vi "Medicao.View.vi"() -> ()   [LabVIEW 2019]
uses:
  Telas.ctl
  <vilib>/Utility/miscctls.llb/LVPositionTypeDef.ctl
  <vilib>/Utility/miscctls.llb/LVPointTypeDef.ctl
  TelaParametrosTeste/VariaveisParametros.vi
  Medicao/VariaveisMedicao.vi
  TelaConfig/Configuracao.Variaveis.vi
  Main/VariaveisTaskMedicao.vi
panel:
  in  "GraphCont":cluster{"X":dbl, "Y":dbl}[](graph)
  out "InfoContinuoRef":T1={"TempRampas"=0.0, "PicoMax"=0.0, "TextUnidMed"="segundos"}
  in  "GraphPontos":cluster{"X":dbl, "Y":dbl}[](array[cluster])
  in  "GraphSenoide":cluster{"X":dbl, "Y":dbl}[](array[cluster])
  out "TimeAquisicao":i32=1000
  out "TimeLastMed":u32
  out "TimeNowMed":u32
  out "Anemometro2":cluster{"X":dbl, "Y":dbl}[](graph)
  out "Anemometro1":cluster{"X":dbl, "Y":dbl}[](graph)
  out "CorrenteAero":cluster{"X":dbl, "Y":dbl}[](graph)
  out "ListaMedicoes":string[][](array[string])
  out "VelocidadeExaustor":cluster{"X":dbl, "Y":dbl}[](graph)
  out "TensaoAero":cluster{"X":dbl, "Y":dbl}[](graph)
  out "TimeInicio":u32
  out "TimeNow":u32
  out "TimeLast":u32
  out "ProximaTela":T2
  in  "Tab":enum32{"Page 1", "Page 2"}(tab)
  in  "QuantMonitora":T3(ring) caption="Tipos de Medição:"
  in  "TabTela":enum32{"Info", "Graph"}(tab)
  out "Text":string
  in  "TaxaTansmissãoDados":dbl caption="Taxa de transmissão de dados:"
  out "UnidadeTaxaTanmissãoDados":string
  out "GeracaoSelecionada":string
  in  "TabOndas":T4(tab)
  out "UnidadeRpm3":string
  in  "InfoContinuo":T1
  out "UnidadeSegundos2":string
  out "UnidadeRpm1":string
  out "UnidadeRpm2":string
  in  "InfoInSenoide":T5
  out "TaxaGeracao":dbl caption="Tempo entre pontos:"
  out "Pontos":dbl[](array[numeric]) caption="Pontos:"
  out "UnidadeSegundos1":string
  out "ListaMedicaoPorta":string[][](table)
  in  "TempoTeste":dbl caption="Tempo do teste:"
  out "UnidadeTempoTeste":string
  in  "MenosVeloz":bool
  in  "MaisVeloz":bool
  out "ValorGraph2":dbl format="%#_5g"
  out "ValorGraph":dbl format="%#_5g"
  out "Graph2":cluster{"X":dbl, "Y":dbl}[](graph)
  out "Graph":cluster{"X":dbl, "Y":dbl}[](graph)
  in  "TipoMedição":u16(ring) caption="Grafico de monitoramento" items=["Velocidade informada"=90, "Velocidade do motor"=91, "Anemômetro 1"=3, "Anemômetro 2"=4, "Corrente AeroGerador"=2, "Tensão AeroGerador"=1]
  in  "TipoMedição2":u16(ring) caption="Grafico de monitoramento" items=["Velocidade informada"=90, "Velocidade do motor"=91, "Anemômetro 1"=3, "Anemômetro 2"=4, "Corrente AeroGerador"=2, "Tensão AeroGerador"=1]
  in  "Play":bool
  in  "Stop":bool
  in  "Voltar":bool
  out "Info":string
  in  "BotaoProximaTela":bool
  in  "VoltarTela":bool
  in  "Salvar":bool
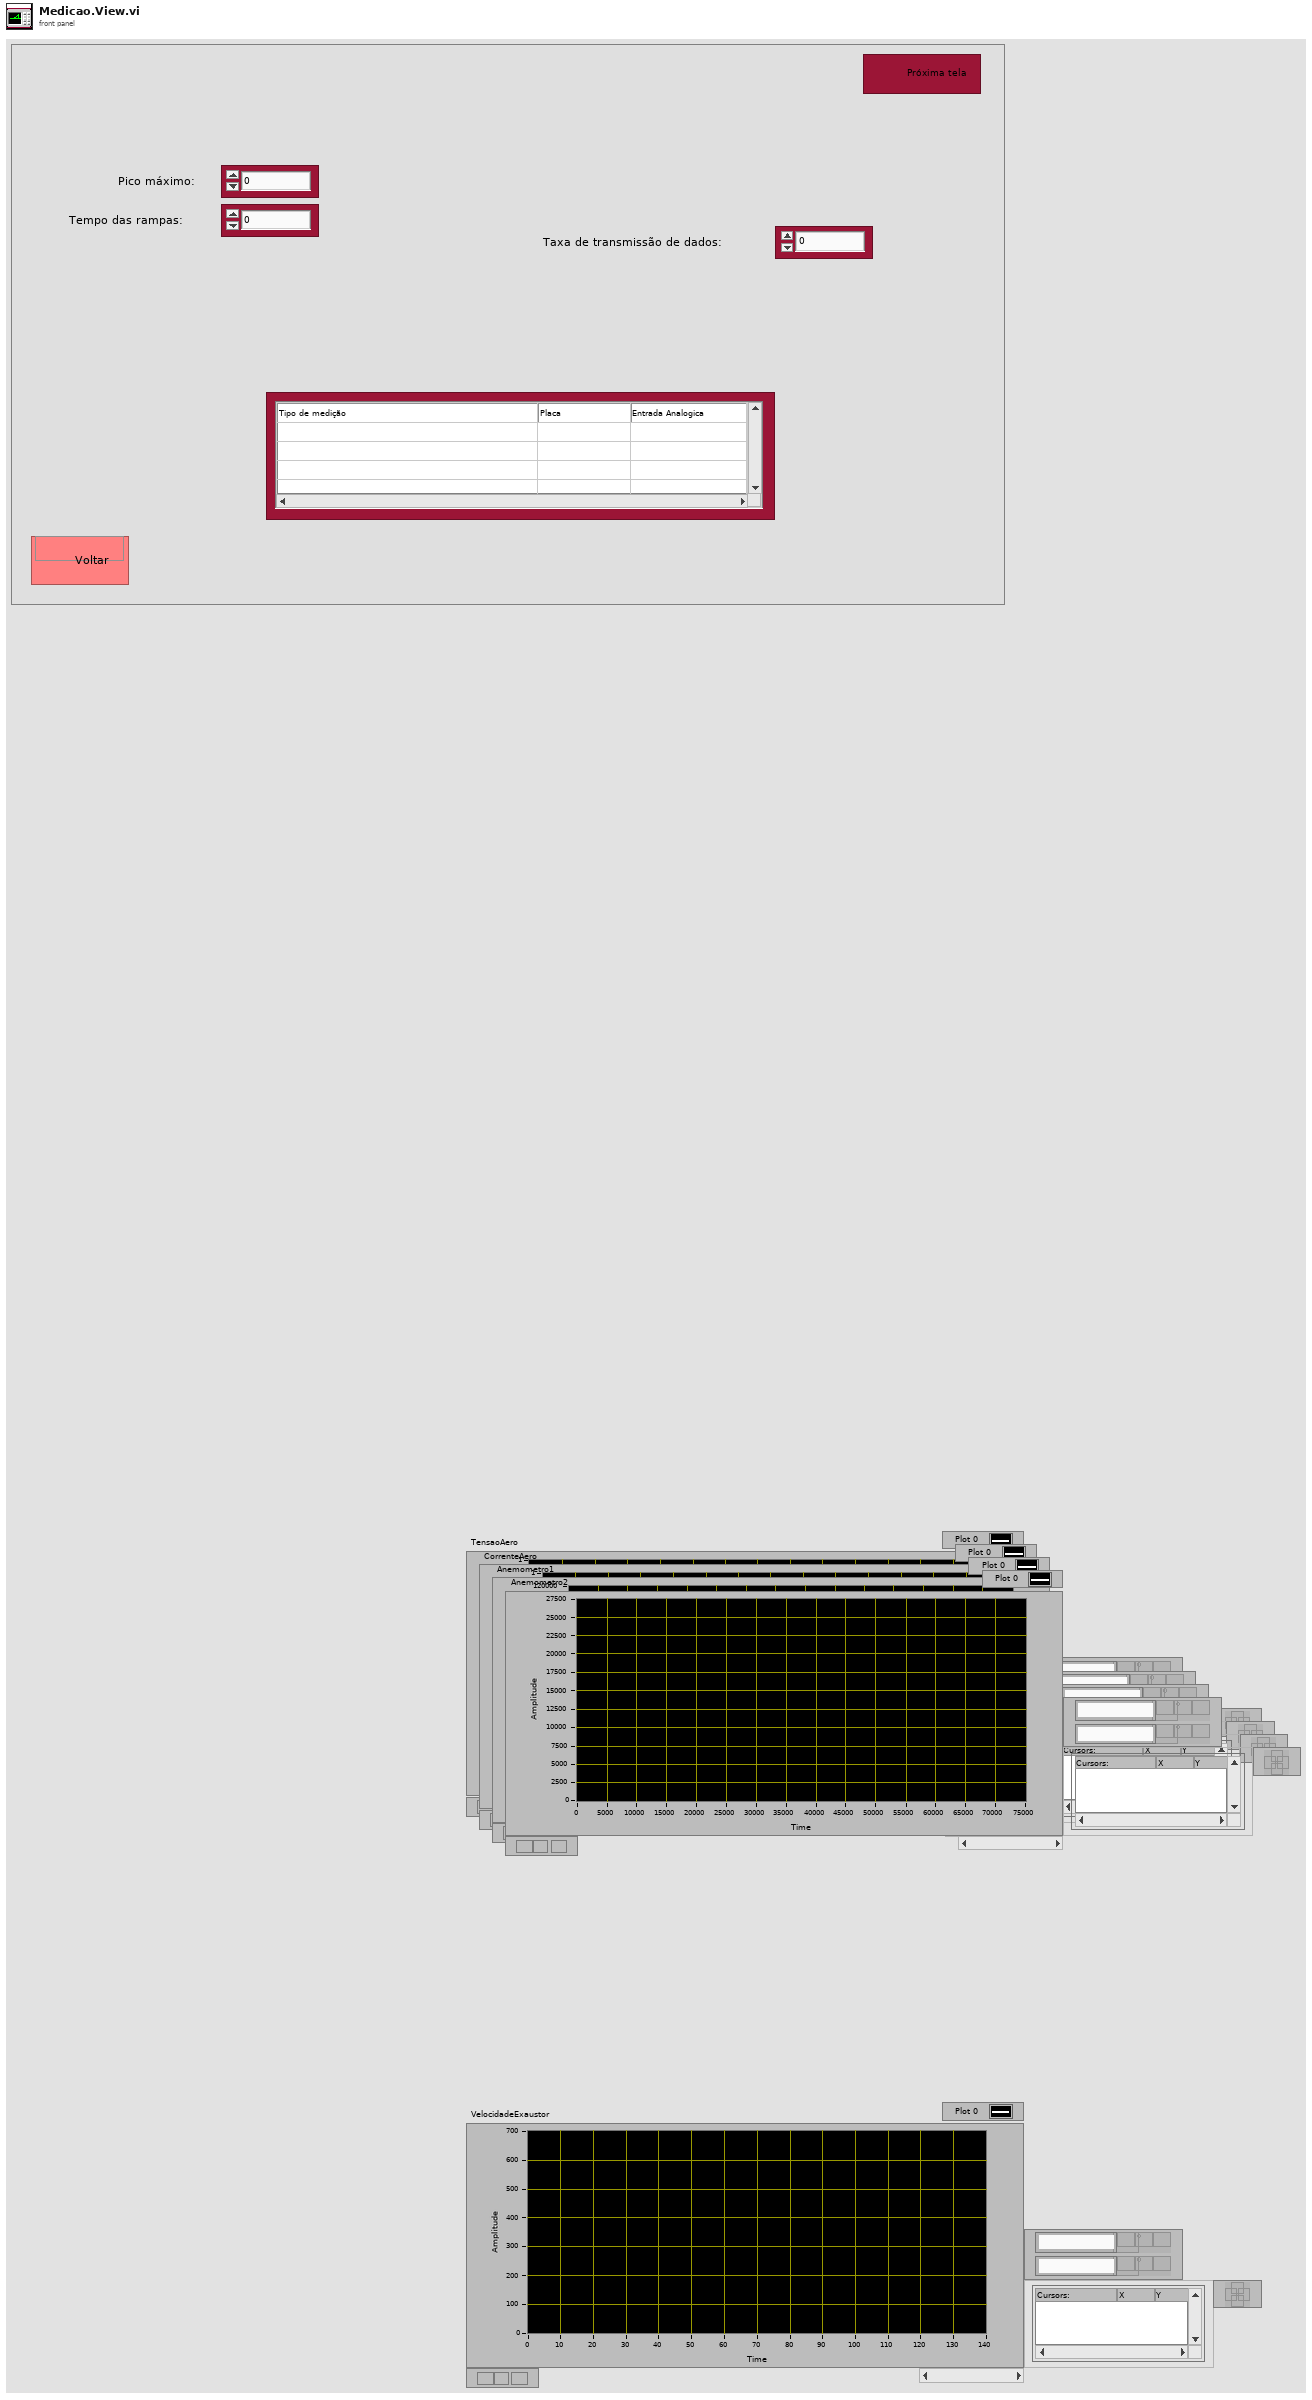
[diagram p1: front panel]
types:
  T1 = cluster{"TempRampas":dbl, "PicoMax":dbl, "TextUnidMed":string}
  T2 = typedef "Telas.ctl" = enum16{"Selecao", "Config", "Medicao", "ParametrosTeste"}
  T3 = enum16{"Monitorar um sinal", "Monitorar dois sinais"}
  T4 = enum32{"Contino", "Senoide", "Pontos", "Quadrada"}
  T5 = cluster{"PicoMax":dbl, "PicoMin":dbl, "RotacaoMinuto":dbl}
  T6 = typedef "LVPositionTypeDef.ctl" = cluster{"Left":i32, "Top":i32}
  T7 = typedef "LVPointTypeDef.ctl" = cluster{"Horizontal":i16, "Vertical":i16}
  T8 = enum16{"OndaContinua", "IniciarRotação", "StatusInversor", "FinalizarRotacao", "OndaSenoide", "OndaPontos", "VelocidadeExaustor"}
  T9 = enum16{"OndaContinua", "IniciarRotação", "StatusInversor", "FinalizarRotacao", "OndaSenoide", "OndaPontos"}
  T10 = enum16{"OndaContinua", "IniciarRotação", "StatusInversor", "FinalizarRotacao", "OndaSenoide", "OndaPontos", "VelocidadeExaustor", "SetInfInversor", "TempoAceleracao", "TempoDesaceleração"}
  T11 = cluster{"PicoRotacaoMax":dbl, "PicoRotacaoMin":dbl, "RotacoesMinuto":dbl}
  T12 = enum16{"None", "Continua", "Senoidal", "Quadrada"}
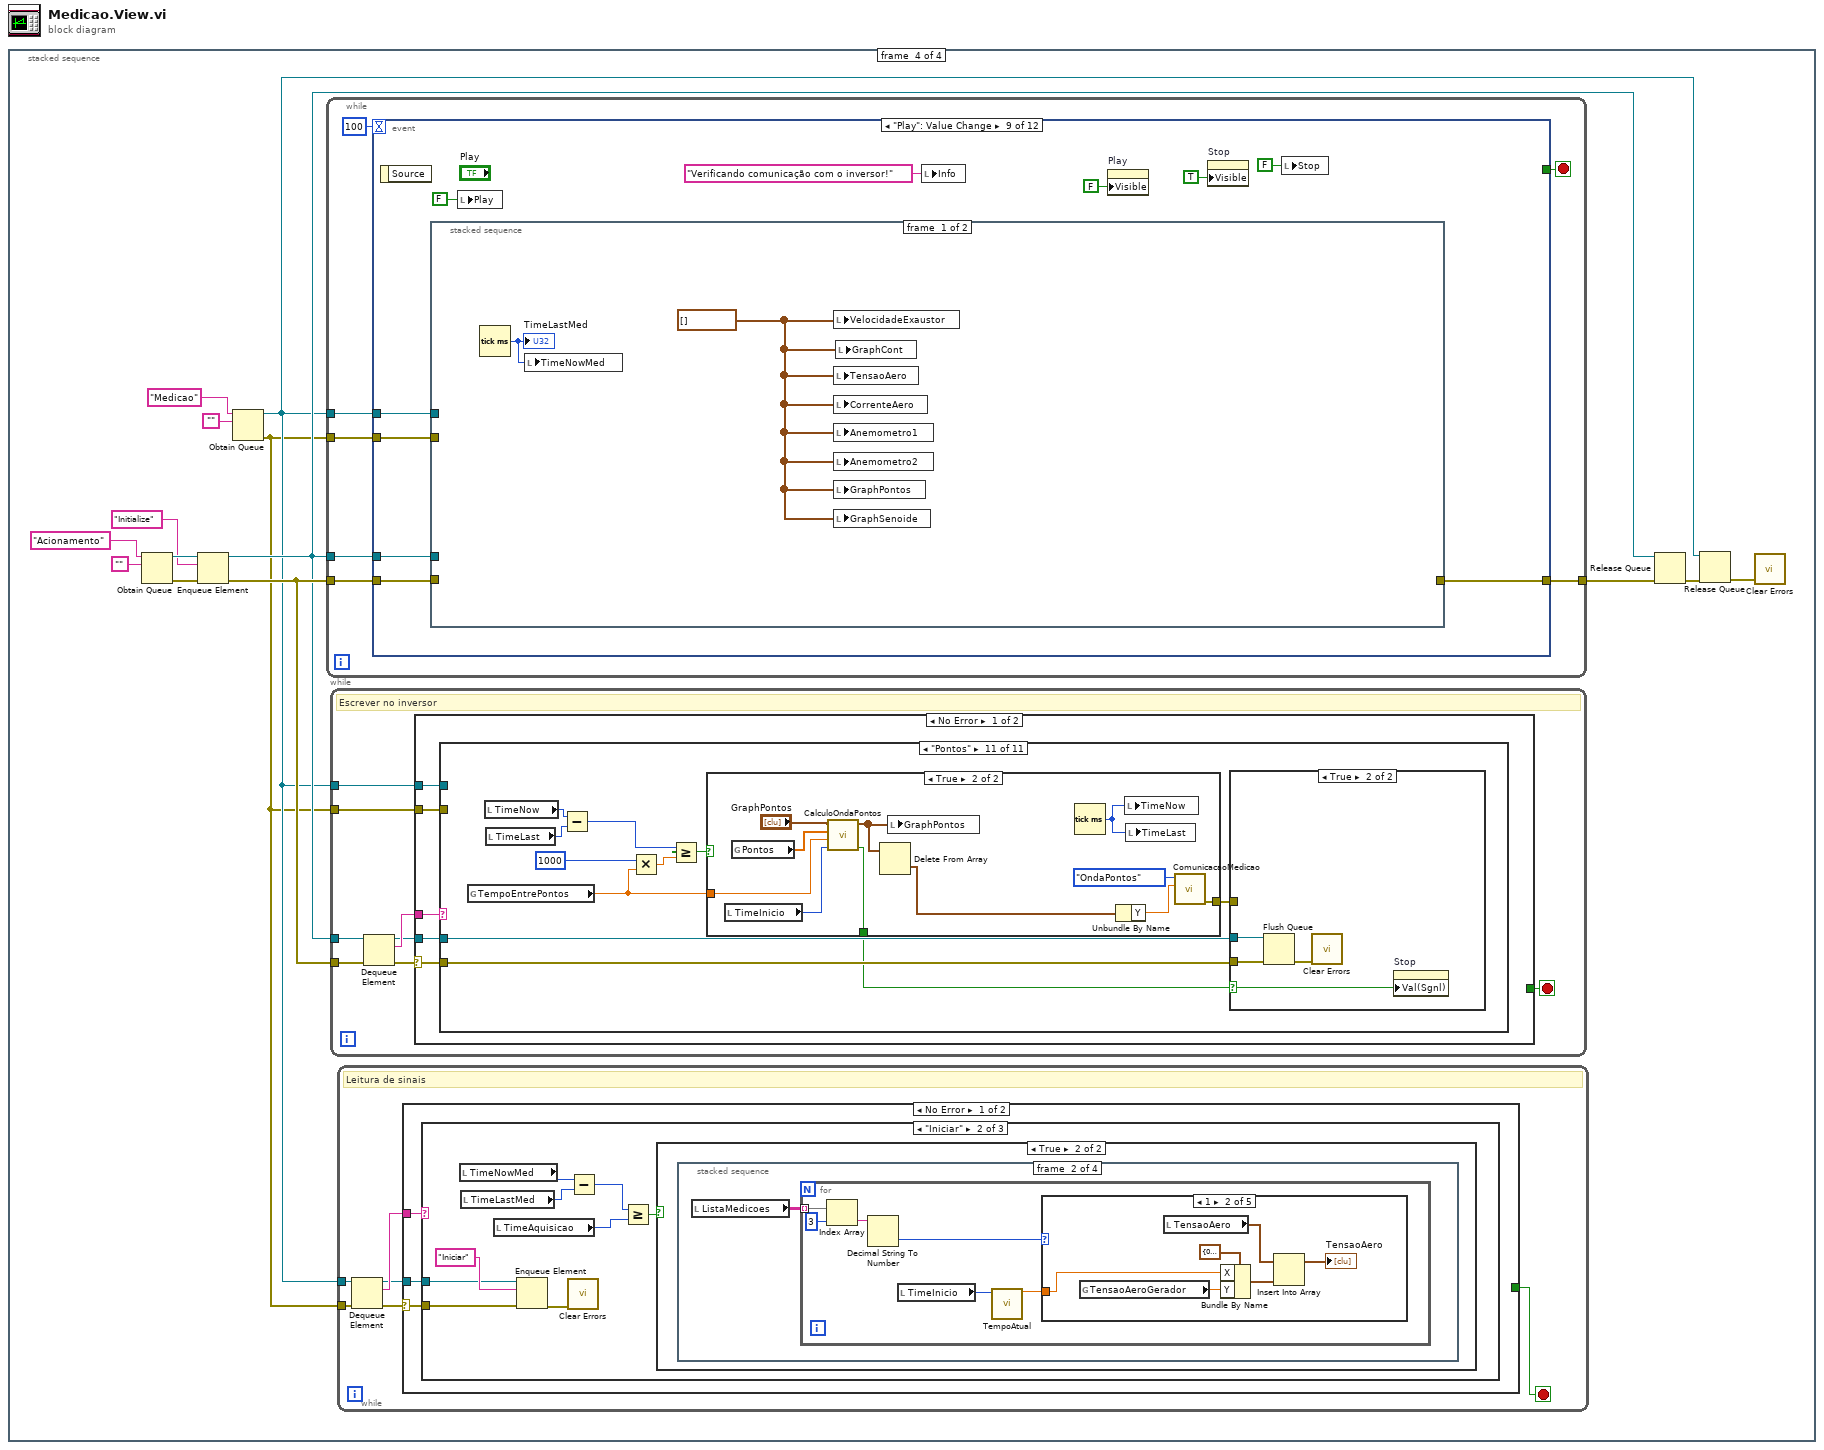
[diagram p0: block diagram]
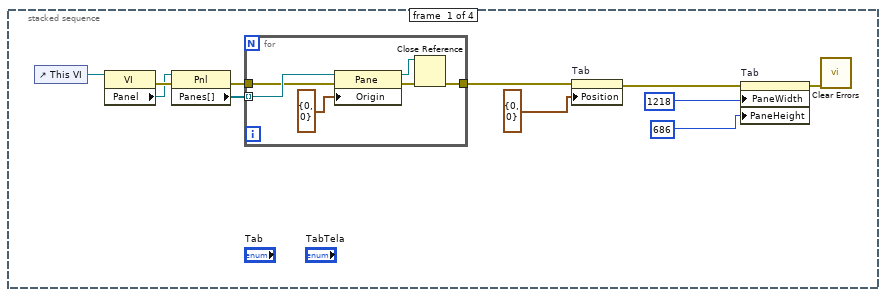
[diagram p2: hidden frame]
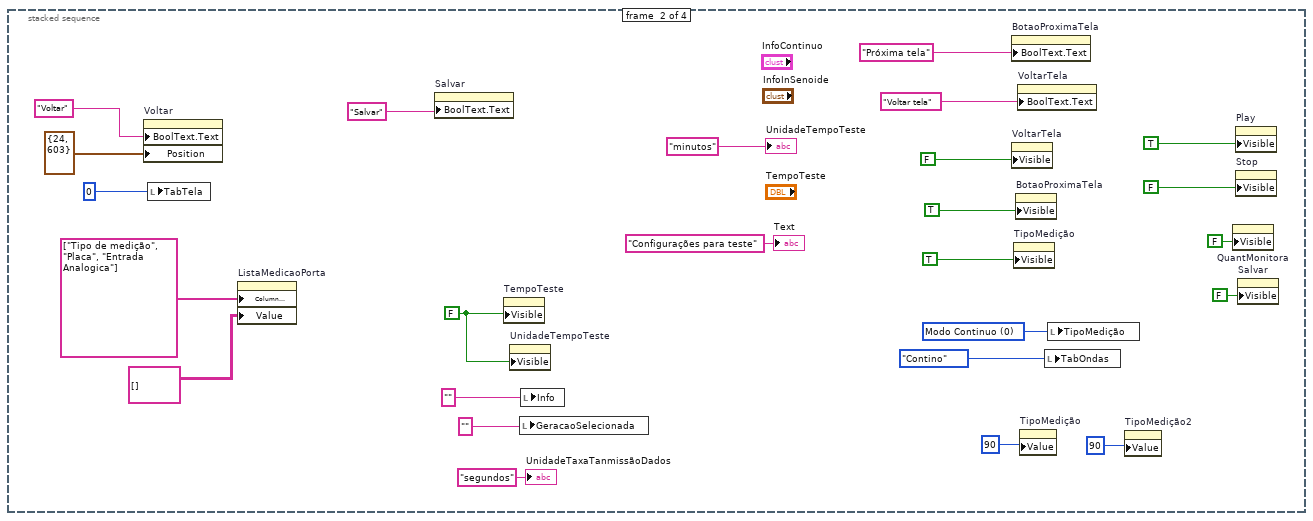
[diagram p3: hidden frame]
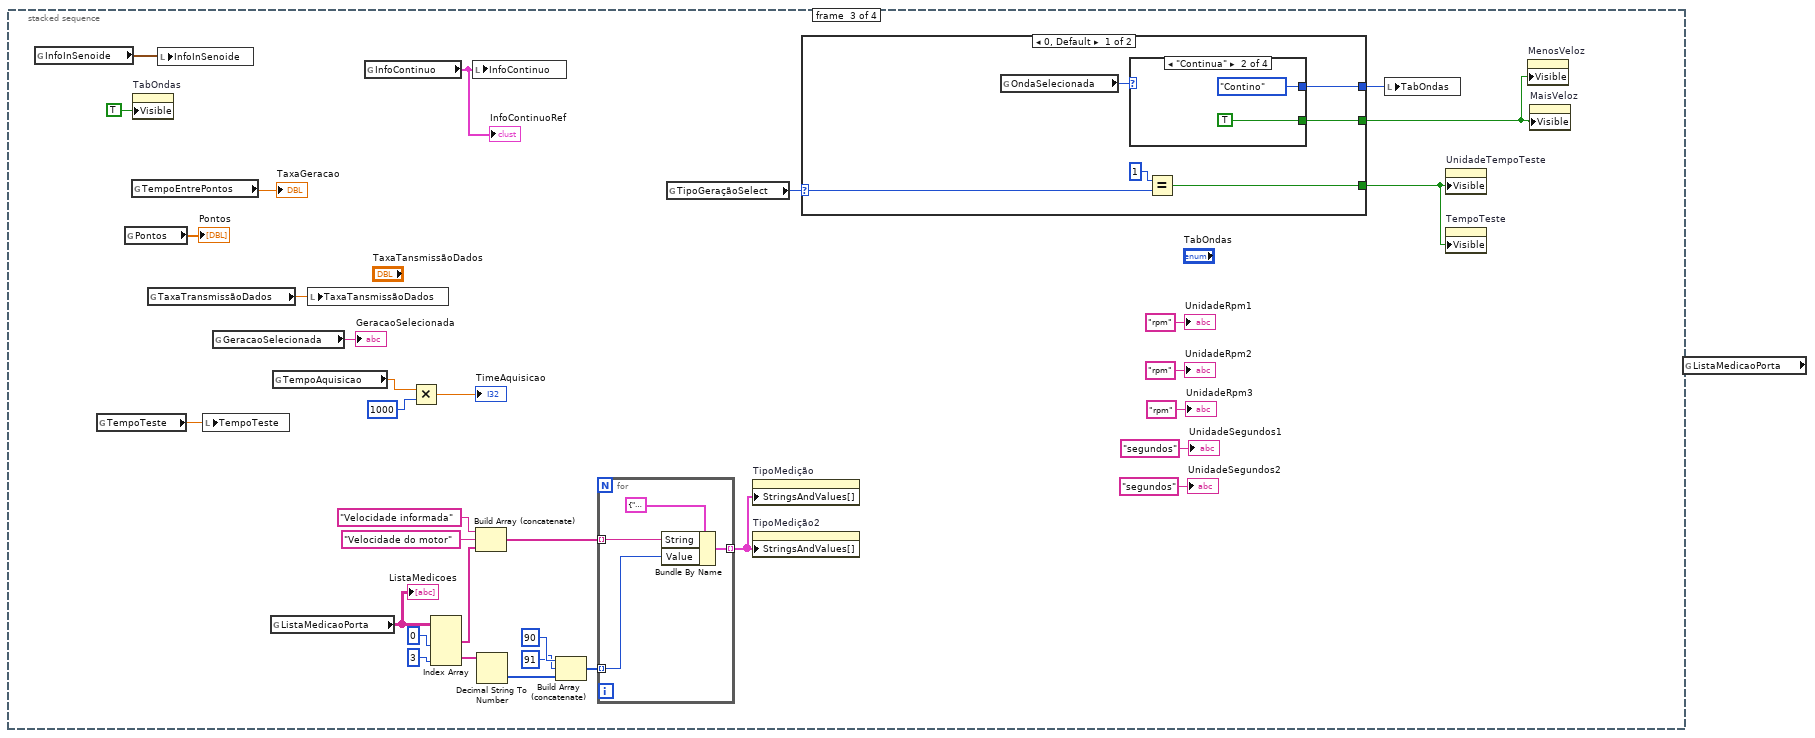
[diagram p4: hidden frame]
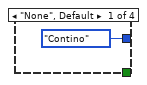
[diagram p5: hidden frame]
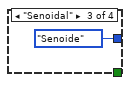
[diagram p6: hidden frame]
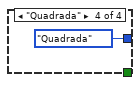
[diagram p7: hidden frame]
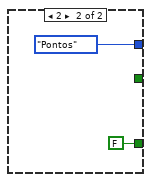
[diagram p8: hidden frame]
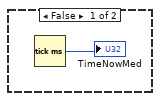
[diagram p10: hidden frame]
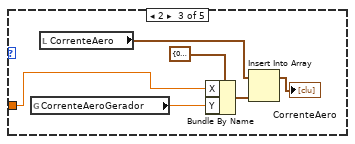
[diagram p13: hidden frame]
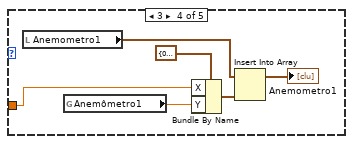
[diagram p14: hidden frame]
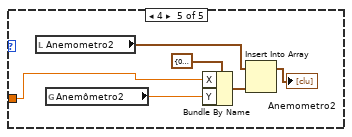
[diagram p15: hidden frame]
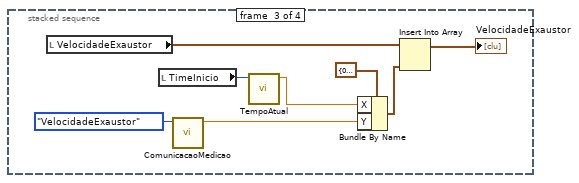
[diagram p16: hidden frame]
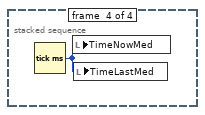
[diagram p17: hidden frame]
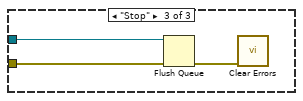
[diagram p18: hidden frame]
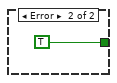
[diagram p19: hidden frame]
diagram:
  n1 = stacked-sequence {
    frame #0 {
      n2 = control-ref of="This VI"() -> (w8:refnum<vi>)
      n3 = property class="VI"(reference=w8) -> (error out=w11:errorcluster, "Panel"=w10:refnum<vi>)  [unwired: 1 in, 1 out]
      n4 = property class="Pnl"(reference=w10, error in=w11) -> (error out=w7:errorcluster, "Panes[]"=w9:refnum<vi>[])  [unwired: 1 out]
      n5 = for {
        tunnel: w9 -> [w17] mode=indexing
        tunnel: w7 -> [w13]
        tunnel: [w12] -> w6
        n6 = property class="Pane"(reference=w17, error in=w13, "Origin"=T7 {"Horizontal"=0, "Vertical"=0}) -> (reference out=w14:refnum<vi>, error out=w15:errorcluster)
        n7 = Close Reference(reference=w14, error in (no error)=w15) -> (error out=w12:errorcluster)
      }
      n8 = property on="Tab" class="TabCtl (strict)"(error in=w6, "Position"=T6 {"Left"=0, "Top"=0}) -> (error out=w5:errorcluster)  [unwired: 1 in, 1 out]
      n9 = property on="Tab" class="TabCtl (strict)"(error in=w5, "PaneWidth"=u32 1218 ("Tab Control Pane Dimension:Width"), "PaneHeight"=u32 686 ("Tab Control Pane Dimension:Height")) -> (error out=w4:errorcluster)  [unwired: 1 in, 1 out]
      n10 = call <vilib>:"Clear Errors.vi"("error in (no error)"=w4) -> ()  [unwired: 5 in, 2 out]
    }
    frame #1 {
      w26 = u16 0 items=["Modo Continuo", "Limitado por tempo", "Ponto por ponto"] ("SelecaoGeracao")
      w30 = FALSE
      n11 = property on="Voltar" class="Bool (strict)"("BoolText.Text"="Voltar" ("Boolean Text.Text"), "Position"=T6 {"Left"=24, "Top"=603}) -> ()  [unwired: 2 in, 2 out]
      n12 = local write "TabTela"(0) -> ()
      n13 = property on="ListaMedicaoPorta" class="Tbl (strict)"("Column Headers[]"=string[] ["Tipo de medição", "Placa", "Entrada Analogica"] ("Column Header Strings[]"), "Value"=string[][] [] ("Item Names")) -> ()  [unwired: 2 in, 2 out]
      n14 = property on="Salvar" class="Bool"("BoolText.Text"="Salvar" ("Boolean Text.Text")) -> ()  [unwired: 2 in, 2 out]
      n15 = property on="TempoTeste" class="DigNum (strict)"("Visible"=w30) -> ()  [unwired: 2 in, 2 out]
      n16 = property on="UnidadeTempoTeste" class="Str"("Visible"=w30) -> ()  [unwired: 2 in, 2 out]
      n17 = local write "GeracaoSelecionada"("" ("GeracaoSelecionada")) -> ()
      n18 = local write "Info"("" ("InfoConfig")) -> ()
      n19 = property on="BotaoProximaTela" class="Bool"("BoolText.Text"="Próxima tela" ("Boolean Text.Text")) -> ()  [unwired: 2 in, 2 out]
      n20 = property on="VoltarTela" class="Bool"("Visible"=FALSE) -> ()  [unwired: 2 in, 2 out]
      n21 = property on="TipoMedição" class="Ring (strict)"("Visible"=TRUE) -> ()  [unwired: 2 in, 2 out]
      n22 = property on="BotaoProximaTela" class="Bool"("Visible"=TRUE) -> ()  [unwired: 2 in, 2 out]
      n23 = property on="VoltarTela" class="Bool"("BoolText.Text"="Voltar tela" ("Boolean Text.Text")) -> ()  [unwired: 2 in, 2 out]
      n24 = property on="TipoMedição" class="Ring (strict)"("Value"=90) -> ()  [unwired: 2 in, 2 out]
      n25 = local write "TabOndas"(T4."Contino" ("TabOndas")) -> ()
      n26 = local write "TipoMedição"(w26) -> ()
      n27 = property on="TipoMedição2" class="Ring (strict)"("Value"=90) -> ()  [unwired: 2 in, 2 out]
      n28 = property on="QuantMonitora" class="Enum (strict)"("Visible"=FALSE) -> ()  [unwired: 2 in, 2 out]
      n29 = property on="Play" class="Bool (strict)"("Visible"=TRUE) -> ()  [unwired: 2 in, 2 out]
      n30 = property on="Stop" class="Bool (strict)"("Visible"=FALSE) -> ()  [unwired: 2 in, 2 out]
      n31 = property on="Salvar" class="Bool"("Visible"=FALSE) -> ()  [unwired: 2 in, 2 out]
      "UnidadeTempoTeste" <- "minutos" ("UnidadeTempoTeste")
      "UnidadeTaxaTanmissãoDados" <- "segundos" ("UnidadeTaxaTanmissãoDados")
      "Text" <- "Configurações para teste" ("String")
    }
    frame #2 {
      n32 = global read "VariaveisParametros.vi" "InfoInSenoide"() -> (w62:T11)
      n33 = global read "VariaveisParametros.vi" "TempoTeste"() -> (w72:dbl)
      n34 = global read "VariaveisParametros.vi" "Pontos"() -> (→"Pontos":dbl[])
      n35 = global read "VariaveisParametros.vi" "TempoEntrePontos"() -> (→"TaxaGeracao":dbl)
      n36 = property on="TabOndas" class="TabCtl (strict)"("Visible"=TRUE) -> ()  [unwired: 2 in, 2 out]
      n37 = global read "VariaveisParametros.vi" "TaxaTransmissãoDados"() -> (w64:dbl)
      n38 = local write "InfoInSenoide"(w62) -> ()
      n39 = local write "TempoTeste"(w72) -> ()
      n40 = global read "VariaveisParametros.vi" "GeracaoSelecionada"() -> (→"GeracaoSelecionada":string)
      n41 = global read "VariaveisParametros.vi" "ListaMedicaoPorta"() -> (w58:string[][])
      "ListaMedicoes" <- w58
      n42 = global read "VariaveisParametros.vi" "TempoAquisicao"() -> (w67:dbl)
      n43 = local write "TaxaTansmissãoDados"(w64) -> ()
      n44 = global read "VariaveisParametros.vi" "InfoContinuo"() -> (w73:T1)
      "InfoContinuoRef" <- w73
      n45 = Multiply(x=w67, y=1000) -> (x*y=→"TimeAquisicao":dbl)
      n46 = Index Array(array=w58, index (col) #1=0 ("disabled index (col)"), index (col) #2=3 ("index (col)")) -> (element #1=w59:string[], element #2=w57:string[])  [unwired: 2 in]
      n47 = local write "InfoContinuo"(w73) -> ()
      n48 = Build Array (concatenate)("Velocidade informada", "Velocidade do motor", w59) -> (w60:string[])
      n49 = Decimal String To Number(string=w57) -> (number=w56:i32[])  [unwired: 2 in, 1 out]
      n50 = Build Array (concatenate)(90, 91, w56) -> (w55:i32[])
      n51 = for {
        tunnel: w60 -> [w79] mode=indexing
        tunnel: [w78] -> w61 mode=indexing
        tunnel: w55 -> [w77] mode=indexing
        n52 = Bundle By Name(cluster=cluster{"String":string, "Value":u16} {"String"="Modo Continuo", "Value"=0}, "String"=w79, "Value"=w77) -> (w78:cluster{"String":string, "Value":u16})
      }
      n53 = global read "VariaveisParametros.vi" "TipoGeraçãoSelect"() -> (w76:u16)
      n54 = property on="TipoMedição" class="Ring (strict)"("StringsAndValues[]"=w61) -> ()  [unwired: 2 in, 2 out]
      n55 = property on="TipoMedição2" class="Ring (strict)"("StringsAndValues[]"=w61) -> ()  [unwired: 2 in, 2 out]
      n56 = case shown="0, Default" w76 {
        selector: w76 -> [w84 _]
        tunnel: [w85 T4."Pontos" ("TabOndas")] -> w75
        tunnel: [w82 FALSE] -> w63
        tunnel: [w81 _] -> w48
        frame 0, Default {
          n57 = global read "VariaveisParametros.vi" "OndaSelecionada"() -> (w86:T12)
          n58 = case shown="\"Continua\"" w86 {
            tunnel: [T4."Contino" ("TabOndas") T4."Contino" ("TabOndas") T4."Senoide" ("TabOndas") T4."Quadrada" ("TabOndas")] -> w85
            tunnel: [_ TRUE _ _] -> w81
            frame "None", Default {
            }
            frame "Continua" {
            }
            frame "Senoidal" {
            }
            frame "Quadrada" {
            }
          }
          n59 = Equal?(x=u16 1, y=w84) -> (x = y?=w82:bool)
        }
        frame 2 {
        }
      }
      n60 = local write "TabOndas"(w75) -> ()
      n61 = property on="UnidadeTempoTeste" class="Str"("Visible"=w63) -> ()  [unwired: 2 in, 2 out]
      n62 = property on="TempoTeste" class="DigNum (strict)"("Visible"=w63) -> ()  [unwired: 2 in, 2 out]
      n63 = property on="MenosVeloz" class="Bool (strict)"("Visible"=w48) -> ()  [unwired: 2 in, 2 out]
      n64 = property on="MaisVeloz" class="Bool (strict)"("Visible"=w48) -> ()  [unwired: 2 in, 2 out]
      n65 = global read "VariaveisParametros.vi" "ListaMedicaoPorta"() -> (→"ListaMedicaoPorta":string[][])
      "UnidadeRpm3" <- "rpm" ("UnidadeTaxaTanmissãoDados 3")
      "UnidadeRpm2" <- "rpm" ("UnidadeTaxaTanmissãoDados 4")
      "UnidadeRpm1" <- "rpm" ("UnidadeTaxaTanmissãoDados 5")
      "UnidadeSegundos1" <- "segundos" ("UnidadeTaxaTanmissãoDados 6")
      "UnidadeSegundos2" <- "segundos" ("UnidadeTaxaTanmissãoDados 2")
    }
    frame #3 {
      n66 = Obtain Queue(name (unnamed)="Acionamento", element data type="") -> (queue out=w105:refnum<queue>, error out=w106:errorcluster)  [unwired: 3 in, 1 out]
      n67 = Enqueue Element(queue=w105, element="Initialize", error in (no error)=w106) -> (queue out=w100:refnum<queue>, error out=w101:errorcluster)  [unwired: 1 in, 1 out]
      n68 = Obtain Queue(name (unnamed)="Medicao", element data type="") -> (queue out=w95:refnum<queue>, error out=w94:errorcluster)  [unwired: 3 in, 1 out]
      n69 = while {
        tunnel: w100 -> [w401]
        tunnel: [w400] -> w102
        tunnel: w101 -> [w399]
        tunnel: w95 -> [w398]
        tunnel: w94 -> [w397]
        stop <- w402 stop-if-true
        n70 = event shown="[8] \"Play\": Value Change" {
          selector: _ -> [_ _ _ _ _ _ _ _ _ _ _ _]
          dyn-events: _ -> [_ _ _ _ _ _ _ _ _ _ _ _]
          timeout: 100 -> [_ _ _ _ _ _ _ _ _ _ _ _]
          tunnel: [FALSE TRUE _ _ _ _ _ _ _ _ _ _] -> w402
          tunnel: w401 -> [_ _ _ _ _ _ _ _ w532 w581 w599 w619]
          tunnel: [w404 _ _ _ _ _ _ _ w534 _ w598 w618] -> w400
          tunnel: w399 -> [w404 _ _ _ _ _ _ _ w533 w580 w600 w620]
          tunnel: w398 -> [_ _ _ _ _ _ _ _ w529 _ _ _]
          tunnel: w397 -> [_ _ _ _ _ _ _ _ w530 _ _ _]
          event Timeout {
            n71 = event-data() -> ()  [unwired: 1 in, 3 out]
            n72 = local read "TabTela"() -> (w405:enum32{"Info", "Graph"})
            n73 = case shown="\"Graph\"" w405 {
              frame Default {
              }
              frame "Graph" {
                n74 = property on="TipoMedição" class="Ring (strict)"() -> ("Value"=w439:u16)  [unwired: 2 in, 2 out]
                n75 = case shown="3" w439 {
                  tunnel: [cluster{"X":dbl, "Y":dbl}[] [] ("OndaCont") w444 w454 w456 w458 w460 w462] -> w437
                  tunnel: ["" w442 "RPM" "Volts" "Ampere" "Velocidade (m/s)" "Velocidade (m/s)"] -> w438
                  frame Default {
                  }
                  frame 90 {
                    n76 = local read "TabOndas"() -> (w443:T4)
                    n77 = case shown="\"Senoide\"" w443 {
                      tunnel: [cluster{"X":dbl, "Y":dbl}[] [] ("OndaCont") w447 w450 w452] -> w444
                      tunnel: ["" "RPM" "RPM" "RPM"] -> w442
                      frame Default {
                      }
                      frame "Contino" {
                        n78 = local read "VelocidadeExaustor"() -> (w447:cluster{"X":dbl, "Y":dbl}[])
                      }
                      frame "Senoide" {
                        n79 = local read "GraphSenoide"() -> (w450:cluster{"X":dbl, "Y":dbl}[])
                      }
                      frame "Pontos" {
                        n80 = local read "GraphPontos"() -> (w452:cluster{"X":dbl, "Y":dbl}[])
                      }
                    }
                  }
                  frame 91 {
                    n81 = local read "VelocidadeExaustor"() -> (w454:cluster{"X":dbl, "Y":dbl}[])
                  }
                  frame 1 {
                    n82 = local read "TensaoAero"() -> (w456:cluster{"X":dbl, "Y":dbl}[])
                  }
                  frame 2 {
                    n83 = local read "CorrenteAero"() -> (w458:cluster{"X":dbl, "Y":dbl}[])
                  }
                  frame 3 {
                    n84 = local read "Anemometro1"() -> (w460:cluster{"X":dbl, "Y":dbl}[])
                  }
                  frame 4 {
                    n85 = local read "Anemometro2"() -> (w462:cluster{"X":dbl, "Y":dbl}[])
                  }
                }
                "Graph" <- w437
                n86 = property on="Graph" class="XYGraph (strict)"("YScale.NameLbl.Text"=w438) -> ()  [unwired: 2 in, 2 out]
                n87 = Delete From Array(array=w437) -> (deleted portion=w436:cluster{"X":dbl, "Y":dbl})  [unwired: 2 in, 1 out]
                n88 = Unbundle By Name(w436) -> ("Y"=→"ValorGraph":dbl)
              }
            }
            n89 = case shown="\"Graph\"" w405 {
              frame Default {
              }
              frame "Graph" {
                n90 = property on="TipoMedição2" class="Ring (strict)"() -> ("Value"=w410:u16)  [unwired: 2 in, 2 out]
                n91 = case shown="4" w410 {
                  tunnel: [cluster{"X":dbl, "Y":dbl}[] [] ("OndaCont") w416 w426 w428 w430 w432 w434] -> w409
                  tunnel: ["" w414 "RPM" "Volts" "Ampere" "Velocidade (m/s)" "Velocidade (m/s)"] -> w408
                  frame Default {
                  }
                  frame 90 {
                    n92 = local read "TabOndas"() -> (w415:T4)
                    n93 = case shown="\"Senoide\"" w415 {
                      tunnel: [cluster{"X":dbl, "Y":dbl}[] [] ("OndaCont") w419 w422 w424] -> w416
                      tunnel: ["" "RPM" "RPM" "RPM"] -> w414
                      frame Default {
                      }
                      frame "Contino" {
                        n94 = local read "VelocidadeExaustor"() -> (w419:cluster{"X":dbl, "Y":dbl}[])
                      }
                      frame "Senoide" {
                        n95 = local read "GraphSenoide"() -> (w422:cluster{"X":dbl, "Y":dbl}[])
                      }
                      frame "Pontos" {
                        n96 = local read "GraphPontos"() -> (w424:cluster{"X":dbl, "Y":dbl}[])
                      }
                    }
                  }
                  frame 91 {
                    n97 = local read "VelocidadeExaustor"() -> (w426:cluster{"X":dbl, "Y":dbl}[])
                  }
                  frame 1 {
                    n98 = local read "TensaoAero"() -> (w428:cluster{"X":dbl, "Y":dbl}[])
                  }
                  frame 2 {
                    n99 = local read "CorrenteAero"() -> (w430:cluster{"X":dbl, "Y":dbl}[])
                  }
                  frame 3 {
                    n100 = local read "Anemometro1"() -> (w432:cluster{"X":dbl, "Y":dbl}[])
                  }
                  frame 4 {
                    n101 = local read "Anemometro2"() -> (w434:cluster{"X":dbl, "Y":dbl}[])
                  }
                }
                "Graph2" <- w409
                n102 = Delete From Array(array=w409) -> (deleted portion=w411:cluster{"X":dbl, "Y":dbl})  [unwired: 2 in, 1 out]
                n103 = property on="Graph2" class="XYGraph (strict)"("YScale.NameLbl.Text"=w408) -> ()  [unwired: 2 in, 2 out]
                n104 = Unbundle By Name(w411) -> ("Y"=→"ValorGraph2":dbl)
              }
            }
          }
          event "Voltar": Value Change {
            n105 = event-data() -> ()  [unwired: 1 in, 6 out]
            n106 = local write "Voltar"(FALSE ("VoltarButton")) -> ()
            n107 = local write "TabTela"(enum32{"Info", "Graph"}."Info" ("TabTela")) -> ()
            "ProximaTela" <- Telas."Selecao" ("NextScreen")
          }
          event "Salvar": Value Change {
            n108 = event-data() -> ()  [unwired: 1 in, 1 out]
            n109 = stacked-sequence {
              seq-local: [w469 _] -> [_ w482]
              frame #0 {
                # "Verifica se o campo esta preenchido corretamente"
                n110 = for {
                  N: 20 -> [_]
                  tunnel: [w470] -> w468 mode=indexing
                  i -> [w471]
                  n111 = case shown="1" w471 {
                    tunnel: [TRUE TRUE] -> w470
                    frame 0, Default {
                    }
                    frame 1 {
                      n112 = local read "VelocidadeExaustor"() -> (w474:cluster{"X":dbl, "Y":dbl}[])
                      n113 = local read "GraphPontos"() -> (w480:cluster{"X":dbl, "Y":dbl}[])
                      n114 = local read "GraphSenoide"() -> (w479:cluster{"X":dbl, "Y":dbl}[])
                      n115 = global write "VariaveisMedicao.vi" "VelocidadeExaustor"(w474) -> ()
                      n116 = global write "VariaveisMedicao.vi" "GraphSenoide"(w479) -> ()
                      n117 = global write "VariaveisMedicao.vi" "GraphPontos"(w480) -> ()
                      n118 = global write "VariaveisMedicao.vi" "OndaCont"("GraphCont") -> ()
                      n119 = local read "TensaoAero"() -> (w478:cluster{"X":dbl, "Y":dbl}[])
                      n120 = local read "CorrenteAero"() -> (w477:cluster{"X":dbl, "Y":dbl}[])
                      n121 = local read "Anemometro1"() -> (w476:cluster{"X":dbl, "Y":dbl}[])
                      n122 = local read "Anemometro2"() -> (w475:cluster{"X":dbl, "Y":dbl}[])
                      n123 = global write "VariaveisMedicao.vi" "Anemometro1"(w476) -> ()
                      n124 = global write "VariaveisMedicao.vi" "Anemometro1"(w475) -> ()
                      n125 = global write "VariaveisMedicao.vi" "CorrenteAero"(w477) -> ()
                      n126 = global write "VariaveisMedicao.vi" "TensaoAero"(w478) -> ()
                    }
                  }
                }
                n127 = And Array Elements(Boolean array=w468) -> (logical AND=w469:bool)
              }
              frame #1 {
                n128 = case shown="True" w482 {
                  frame False {
                    # "Algo não esta preenchido corretamente"
                    "Info" <- "" ("InfoConfig")
                  }
                  frame True {
                    # "Preenchimento correto dos campos"
                    n129 = call "SalvarInformacoesRelatorio.vi"() -> ("error out"=w485:errorcluster, "NomeDocumento"=w484:string)  [unwired: 10 in]
                    n130 = case shown="No Error" w485 {
                      selector: w485 -> [w489 _]
                      tunnel: [w490 "Erro ao salvar as variavies" ("InfoConfig")] -> w486
                      tunnel: w484 -> [w488 _]
                      frame No Error {
                        n131 = call "Geracao_Excel.vi"("error in (no error)"=w489, "FileName"=w488) -> ("error out"=w487:errorcluster)  [unwired: 9 in]
                        n132 = case shown="Error .." w487 {
                          tunnel: ["Informações salvas e gerado relatório" ("InfoConfig") "Informações salvas e erro ao gerar o relatório" ("InfoConfig")] -> w490
                          frame No Error {
                          }
                          frame Error {
                          }
                        }
                      }
                      frame Error {
                      }
                    }
                    n133 = local write "Info"(w486) -> ()
                  }
                }
              }
            }
          }
          event "BotaoProximaTela": Value Change {
            n134 = event-data() -> ()  [unwired: 1 in, 1 out]
            n135 = local read "TabTela"() -> (w499:enum32{"Info", "Graph"})
            n136 = Increment(x=w499) -> (x+1=w495:enum32{"Info", "Graph"})
            n137 = case shown="\"Info\"" w495 {
              tunnel: [TRUE FALSE TRUE] -> w498
              tunnel: [TRUE TRUE FALSE] -> w497
              tunnel: [TRUE FALSE TRUE] -> w496
              frame Default {
              }
              frame "Info" {
                w503 = u16 0 ("Value (Signaling)")
                n138 = property on="TipoMedição" class="Ring (strict)"("Val(Sgnl)"=w503) -> ()  [unwired: 2 in, 2 out]
                n139 = property on="TipoMedição2" class="Ring (strict)"("Value"=w503) -> ()  [unwired: 2 in, 2 out]
              }
              frame "Graph" {
              }
            }
            n140 = local write "TabTela"(w495) -> ()
            n141 = property on="Salvar" class="Bool"("Visible"=TRUE) -> ()  [unwired: 2 in, 2 out]
            n142 = property on="VoltarTela" class="Bool"("Visible"=w498) -> ()  [unwired: 2 in, 2 out]
            n143 = property on="ProximaTela" class="Bool"("Visible"=w497) -> ()  [unwired: 2 in, 2 out]
            n144 = property on="TipoMedição" class="Ring (strict)"("Visible"=w496) -> ()  [unwired: 2 in, 2 out]
          }
          event "VoltarTela": Value Change {
            n145 = event-data() -> ()  [unwired: 1 in, 6 out]
            n146 = local read "TabTela"() -> (w515:enum32{"Info", "Graph"})
            n147 = property on="Salvar" class="Bool"("Visible"=FALSE) -> ()  [unwired: 2 in, 2 out]
            n148 = Decrement(x=w515) -> (x-1=w511:enum32{"Info", "Graph"})
            n149 = local write "TabTela"(w511) -> ()
            n150 = case shown="Default" w511 {
              tunnel: [TRUE FALSE TRUE] -> w514
              tunnel: [TRUE TRUE FALSE] -> w513
              tunnel: [TRUE FALSE TRUE] -> w512
              frame Default {
              }
              frame "Info" {
              }
              frame "Graph" {
              }
            }
            n151 = property on="VoltarTela" class="Bool"("Visible"=w514) -> ()  [unwired: 2 in, 2 out]
            n152 = property on="ProximaTela" class="Bool"("Visible"=w513) -> ()  [unwired: 2 in, 2 out]
            n153 = property on="TipoMedição" class="Ring (strict)"("Visible"=w512) -> ()  [unwired: 2 in, 2 out]
          }
          event "TipoMedição": Value Change {
            n154 = event-data() -> ()  [unwired: 1 in, 1 out]
          }
          event "TipoMedição2": Value Change {
            n155 = event-data() -> ()  [unwired: 1 in, 1 out]
          }
          event "QuantMonitora": Value Change {
            n156 = event-data() -> ()  [unwired: 1 in, 6 out]
            n157 = case shown="\"Monitorar dois sinais\"" "QuantMonitora" {
              tunnel: [FALSE TRUE] -> w525
              frame "Monitorar um sinal", Default {
              }
              frame "Monitorar dois sinais" {
              }
            }
            n158 = property on="TipoMedição2" class="Ring (strict)"("Visible"=w525) -> ()  [unwired: 2 in, 2 out]
          }
          event "Play": Value Change {
            n159 = event-data() -> ()  [unwired: 1 in, 1 out]
            n160 = stacked-sequence {
              tunnel: [_ w555] -> w534
              tunnel: w533 -> [_ w554]
              tunnel: w532 -> [_ w553]
              tunnel: w530 -> [_ w551]
              tunnel: w529 -> [_ w550]
              frame #0 {
                w539 = cluster{"X":dbl, "Y":dbl}[] [] ("OndaCont")
                n161 = Tick Count (ms)() -> (millisecond timer value=w540:u32)
                "TimeLastMed" <- w540
                n162 = local write "TimeNowMed"(w540) -> ()
                n163 = local write "VelocidadeExaustor"(w539) -> ()
                n164 = local write "TensaoAero"(w539) -> ()
                n165 = local write "CorrenteAero"(w539) -> ()
                n166 = local write "Anemometro1"(w539) -> ()
                n167 = local write "Anemometro2"(w539) -> ()
                n168 = local write "GraphPontos"(w539) -> ()
                n169 = local write "GraphSenoide"(w539) -> ()
                n170 = local write "GraphCont"(w539) -> ()
              }
              frame #1 {
                n171 = Enqueue Element(queue=w553, element="StatusInversor", error in (no error)=w554) -> (queue out=w545:refnum<queue>, error out=w546:errorcluster)  [unwired: 1 in, 1 out]
                n172 = Enqueue Element(queue=w550, element="Iniciar", error in (no error)=w551) -> (error out=w549:errorcluster)  [unwired: 1 in, 2 out]
                n173 = call <vilib>:"Clear Errors.vi"("error in (no error)"=w549) -> ()  [unwired: 5 in, 2 out]
                n174 = Enqueue Element(queue=w545, element="SetInfoInversor", error in (no error)=w546) -> (queue out=w543:refnum<queue>, error out=w542:errorcluster)  [unwired: 1 in, 1 out]
                n175 = local read "TabOndas"() -> (w548:T4)
                n176 = case shown="\"Contino\", Default" w548 {
                  tunnel: [w561 w571 w578] -> w555
                  tunnel: w543 -> [w563 w570 w577]
                  tunnel: w542 -> [w564 w568 w575]
                  frame "Contino", Default {
                    n177 = Enqueue Element(queue=w563, element="SetRampa", error in (no error)=w564) -> (queue out=w559:refnum<queue>, error out=w558:errorcluster)  [unwired: 1 in, 1 out]
                    n178 = Enqueue Element(queue=w559, element="SetVelocidade", error in (no error)=w558) -> (queue out=w557:refnum<queue>, error out=w556:errorcluster)  [unwired: 1 in, 1 out]
                    n179 = Enqueue Element(queue=w557, element="IniciarRotacao", error in (no error)=w556) -> (error out=w561:errorcluster)  [unwired: 1 in, 2 out]
                  }
                  frame "Senoide" {
                    n180 = Enqueue Element(queue=w570, element="IniciarRotacao", error in (no error)=w568) -> (queue out=w567:refnum<queue>, error out=w566:errorcluster)  [unwired: 1 in, 1 out]
                    n181 = Enqueue Element(queue=w567, element="Senoidal", error in (no error)=w566) -> (error out=w571:errorcluster)  [unwired: 1 in, 2 out]
                  }
                  frame "Pontos" {
                    n182 = Enqueue Element(queue=w577, element="IniciarRotacao", error in (no error)=w575) -> (queue out=w574:refnum<queue>, error out=w573:errorcluster)  [unwired: 1 in, 1 out]
                    n183 = Enqueue Element(queue=w574, element="Pontos", error in (no error)=w573) -> (error out=w578:errorcluster)  [unwired: 1 in, 2 out]
                  }
                }
                n184 = Tick Count (ms)() -> (millisecond timer value=→"TimeInicio":u32)
              }
            }
            n185 = local write "Play"(FALSE ("Stop")) -> ()
            n186 = local write "Info"("Verificando comunicação com o inversor!" ("Info")) -> ()
            n187 = property on="Play" class="Bool (strict)"("Visible"=FALSE) -> ()  [unwired: 2 in, 2 out]
            n188 = property on="Stop" class="Bool (strict)"("Visible"=TRUE) -> ()  [unwired: 2 in, 2 out]
            n189 = local write "Stop"(FALSE ("Stop")) -> ()
          }
          event "Stop": Value Change {
            n190 = event-data() -> ()  [unwired: 1 in, 1 out]
            n191 = local write "Stop"(FALSE ("Play")) -> ()
            n192 = local read "TabOndas"() -> (w582:T4)
            n193 = property on="Play" class="Bool (strict)"("Visible"=TRUE) -> ()  [unwired: 2 in, 2 out]
            n194 = case shown="\"Contino\", Default" w582 {
              tunnel: w580 -> [w590 w594]
              tunnel: w581 -> [w589 w596]
              frame "Contino", Default {
                n195 = Flush Queue(queue=w589, error in (no error)=w590) -> (queue out=w587:refnum<queue>, error out=w588:errorcluster)  [unwired: 1 out]
                n196 = Tick Count (ms)() -> (millisecond timer value=w592:u32)
                n197 = local write "TimeNow"(w592) -> ()
                n198 = local write "TimeLast"(w592) -> ()
                n199 = Enqueue Element(queue=w587, element="FinalizarRotacao", error in (no error)=w588) -> (error out=w591:errorcluster)  [unwired: 1 in, 2 out]
                n200 = call <vilib>:"Clear Errors.vi"("error in (no error)"=w591) -> ()  [unwired: 5 in, 2 out]
              }
              frame "Senoide" {
                n201 = Enqueue Element(queue=w596, element="FinalizarRotacao", error in (no error)=w594) -> (error out=w597:errorcluster)  [unwired: 1 in, 2 out]
                n202 = call <vilib>:"Clear Errors.vi"("error in (no error)"=w597) -> ()  [unwired: 5 in, 2 out]
              }
            }
            n203 = local write "Play"(FALSE ("Play")) -> ()
            n204 = property on="Stop" class="Bool (strict)"("Visible"=FALSE) -> ()  [unwired: 2 in, 2 out]
          }
          event "MaisVeloz": Value Change {
            n205 = event-data() -> ()  [unwired: 1 in, 1 out]
            n206 = local read "TabOndas"() -> (w601:T4)
            n207 = local write "MaisVeloz"(FALSE ("MaisVeloz")) -> ()
            n208 = case shown="\"Contino\"" w601 {
              tunnel: w600 -> [w603 w606]
              tunnel: w599 -> [_ w605]
              tunnel: [w603 w604] -> w598
              frame Default {
              }
              frame "Contino" {
                n209 = flat-sequence {
                  tunnel: w606 -> [w616]
                  tunnel: w605 -> [w615]
                  tunnel: [w614] -> w604
                  frame #0 {
                    n210 = local read "InfoContinuoRef"() -> (w612:T1)
                    n211 = global read "Configuracao.Variaveis.vi" "RotacaoMaxSistema"() -> (w609:dbl)
                    n212 = Unbundle By Name(w612) -> ("PicoMax"=w611:dbl)
                    n213 = Increment(x=w611) -> (x+1=w608:dbl)
                    n214 = Greater Or Equal?(x=w608, y=w609) -> (x >= y?=w610:bool)
                    n215 = Select(t=w609, s=w610, f=w608) -> (s? t:f=w607:dbl)
                    n216 = Bundle By Name(cluster=w612, "PicoMax"=w607) -> (w613:T1)
                    n217 = local write "InfoContinuoRef"(w613) -> ()
                  }
                  frame #1 {
                    n218 = Enqueue Element(queue=w615, element="SetVelocidade", error in (no error)=w616) -> (error out=w614:errorcluster)  [unwired: 1 in, 2 out]
                  }
                }
              }
            }
          }
          event "MenosVeloz": Value Change {
            n219 = event-data() -> ()  [unwired: 1 in, 1 out]
            n220 = local read "TabOndas"() -> (w621:T4)
            n221 = local write "MenosVeloz"(FALSE ("MaisVeloz")) -> ()
            n222 = case shown="\"Contino\"" w621 {
              tunnel: w620 -> [w623 w626]
              tunnel: w619 -> [_ w625]
              tunnel: [w623 w624] -> w618
              frame Default {
              }
              frame "Contino" {
                n223 = flat-sequence {
                  tunnel: w626 -> [w636]
                  tunnel: w625 -> [w635]
                  tunnel: [w634] -> w624
                  frame #0 {
                    w627 = 0.0
                    n224 = local read "InfoContinuoRef"() -> (w632:T1)
                    n225 = Unbundle By Name(w632) -> ("PicoMax"=w631:dbl)
                    n226 = Decrement(x=w631) -> (x-1=w628:dbl)
                    n227 = Less Or Equal?(x=w628, y=w627) -> (x <= y?=w629:bool)
                    n228 = Select(t=w627, s=w629, f=w628) -> (s? t:f=w630:dbl)
                    n229 = Bundle By Name(cluster=w632, "PicoMax"=w630) -> (w633:T1)
                    n230 = local write "InfoContinuoRef"(w633) -> ()
                  }
                  frame #1 {
                    n231 = Enqueue Element(queue=w635, element="SetVelocidade", error in (no error)=w636) -> (error out=w634:errorcluster)  [unwired: 1 in, 2 out]
                  }
                }
              }
            }
          }
        }
      }
      n232 = while {
        tunnel: w101 -> [w177]
        tunnel: w100 -> [w176]
        tunnel: w95 -> [w172]
        tunnel: w94 -> [w171]
        stop <- w174 stop-if-true
        # "Escrever no inversor"
        n233 = Dequeue Element(queue=w176, error in (no error)=w177) -> (queue out=w173:refnum<queue>, element=w175:string, error out=w178:errorcluster)  [unwired: 1 in, 1 out]
        n234 = case shown="No Error" w178 {
          selector: w178 -> [w181 _]
          tunnel: w175 -> [w183 _]
          tunnel: [_ TRUE] -> w174
          tunnel: w173 -> [w182 _]
          tunnel: w172 -> [w180 _]
          tunnel: w171 -> [w179 _]
          frame No Error {
            n235 = case shown="\"Pontos\"" w183 {
              tunnel: w182 -> [_ _ w186 w209 w233 w258 _ _ w295 w315 w363]
              tunnel: w181 -> [_ _ w187 w210 w234 w257 _ _ w296 w316 w364]
              tunnel: w180 -> [_ _ _ _ _ w253 _ _ _ _ _]
              tunnel: w179 -> [_ _ _ _ _ w254 _ _ _ _ _]
              frame Default {
              }
              frame "Initialize" {
                # "Testar a cominicação"
              }
              frame "StatusInversor" {
                n236 = call "SeparaMemoriaStatusMotor.vi"() -> ("error out"=w189:errorcluster)  [unwired: 10 in, 1 out]
                n237 = call "ComunicacaoMedicao.vi"("error in"=w189, "Operação"=T9."StatusInversor") -> ("error out"=w188:errorcluster)  [unwired: 7 in, 2 out]
                n238 = call <vilib>:"Clear Errors.vi"("error in (no error)"=w188) -> ("error out"=w185:errorcluster)  [unwired: 5 in, 1 out]
                n239 = case shown="No Error" w185 {
                  selector: w185 -> [w192 w202]
                  tunnel: w187 -> [_ w197]
                  tunnel: w186 -> [_ w196]
                  frame No Error {
                    n240 = call "AnaliseStatusInversor.vi"("error in"=w192) -> ("InfoStatus"=w191:string)  [unwired: 8 in, 2 out]
                    n241 = local write "Info"(w191) -> ()
                    n242 = Wait (ms)(milliseconds to wait=u32 1000) -> ()  [unwired: 1 out]
                  }
                  frame Error {
                    n243 = Unbundle By Name(w202) -> ("source"=w200:string)
                    n244 = Concatenate Strings("Erro na Comunicação com o inversor" ("Info"), "\r", w200) -> (w199:string)
                    n245 = local write "Info"(w199) -> ()
                    n246 = disable-structure shown="Disabled" {
                      disable-tunnel: w197 -> [w205 _]
                      disable-tunnel: w196 -> [w204 _]
                      frame Disabled {
                        n247 = Flush Queue(queue=w204, error in (no error)=w205) -> (error out=w203:errorcluster)  [unwired: 2 out]
                        n248 = call <vilib>:"Clear Errors.vi"("error in (no error)"=w203) -> ()  [unwired: 5 in, 2 out]
                      }
                      frame Enabled {
                      }
                    }
                    n249 = property on="Play" class="Bool (strict)"("Visible"=TRUE) -> ()  [unwired: 2 in, 2 out]
                    n250 = local write "Play"(FALSE ("Play")) -> ()
                    n251 = property on="Stop" class="Bool (strict)"("Visible"=FALSE) -> ()  [unwired: 2 in, 2 out]
                  }
                }
              }
              frame "SetInfoInversor" {
                n252 = call "SeparaMemoriaSetDadosInversor.vi"() -> ("error out"=w206:errorcluster)  [unwired: 10 in, 1 out]
                n253 = call "ComunicacaoMedicao.vi"("error in"=w206, "Operação"=T9."StatusInversor") -> ("error out"=w211:errorcluster)  [unwired: 7 in, 2 out]
                n254 = call <vilib>:"Clear Errors.vi"("error in (no error)"=w211) -> ("error out"=w208:errorcluster)  [unwired: 5 in, 1 out]
                n255 = case shown="No Error" w208 {
                  selector: w208 -> [w214 w224]
                  tunnel: w210 -> [_ w219]
                  tunnel: w209 -> [_ w218]
                  frame No Error {
                    n256 = call "AnaliseStatusInversor.vi"("error in"=w214) -> ("InfoStatus"=w213:string)  [unwired: 8 in, 2 out]
                    n257 = local write "Info"(w213) -> ()
                    n258 = Wait (ms)(milliseconds to wait=u32 1000) -> ()  [unwired: 1 out]
                  }
                  frame Error {
                    n259 = Unbundle By Name(w224) -> ("source"=w222:string)
                    n260 = Concatenate Strings("Erro na Comunicação com o inversor" ("Info"), "\r", w222) -> (w221:string)
                    n261 = local write "Info"(w221) -> ()
                    n262 = disable-structure shown="Disabled" {
                      disable-tunnel: w219 -> [w227 _]
                      disable-tunnel: w218 -> [w226 _]
                      frame Disabled {
                        n263 = Flush Queue(queue=w226, error in (no error)=w227) -> (error out=w225:errorcluster)  [unwired: 2 out]
                        n264 = call <vilib>:"Clear Errors.vi"("error in (no error)"=w225) -> ()  [unwired: 5 in, 2 out]
                      }
                      frame Enabled {
                      }
                    }
                    n265 = property on="Play" class="Bool (strict)"("Visible"=TRUE) -> ()  [unwired: 2 in, 2 out]
                    n266 = local write "Play"(FALSE ("Play")) -> ()
                    n267 = property on="Stop" class="Bool (strict)"("Visible"=FALSE) -> ()  [unwired: 2 in, 2 out]
                  }
                }
              }
              frame "IniciarRotacao" {
                n268 = call "SeparaMemoriaPlayRotacao.vi"("Acionamento"=enum16{"Play", "Stop"}."Play") -> ("error out"=w232:errorcluster, "InfoStatus"=w230:string)  [unwired: 8 in, 1 out]
                n269 = call "ComunicacaoMedicao.vi"("error in"=w232, "Operação"=T9."IniciarRotação") -> ("error out"=w235:errorcluster)  [unwired: 7 in, 2 out]
                n270 = call <vilib>:"Clear Errors.vi"("error in (no error)"=w235) -> ("error out"=w229:errorcluster)  [unwired: 5 in, 1 out]
                n271 = case shown="No Error" w229 {
                  selector: w229 -> [_ w248]
                  tunnel: w234 -> [_ w243]
                  tunnel: w233 -> [_ w242]
                  tunnel: w230 -> [w237 _]
                  frame No Error {
                    n272 = local write "Info"(w237) -> ()
                    n273 = Tick Count (ms)() -> (millisecond timer value=→"TimeLast" →"TimeNow":u32)
                  }
                  frame Error {
                    n274 = Unbundle By Name(w248) -> ("source"=w246:string)
                    n275 = Concatenate Strings("Erro na Comunicação com o inversor" ("Info"), "\r", w246) -> (w245:string)
                    n276 = local write "Info"(w245) -> ()
                    n277 = Flush Queue(queue=w242, error in (no error)=w243) -> (error out=w241:errorcluster)  [unwired: 2 out]
                    n278 = call <vilib>:"Clear Errors.vi"("error in (no error)"=w241) -> ()  [unwired: 5 in, 2 out]
                    n279 = property on="Play" class="Bool (strict)"("Visible"=TRUE) -> ()  [unwired: 2 in, 2 out]
                    n280 = local write "Play"(FALSE ("Play")) -> ()
                    n281 = property on="Stop" class="Bool (strict)"("Visible"=FALSE) -> ()  [unwired: 2 in, 2 out]
                  }
                }
              }
              frame "FinalizarRotacao" {
                n282 = call "SeparaMemoriaPlayRotacao.vi"("Acionamento"=enum16{"Play", "Stop"}."Stop") -> ("error out"=w262:errorcluster, "InfoStatus"=w260:string)  [unwired: 8 in, 1 out]
                n283 = Flush Queue(queue=w253, error in (no error)=w254) -> (queue out=w250:refnum<queue>, error out=w255:errorcluster)  [unwired: 1 out]
                n284 = Flush Queue(queue=w258, error in (no error)=w257) -> (error out=w259:errorcluster)  [unwired: 2 out]
                n285 = call <vilib>:"Clear Errors.vi"("error in (no error)"=w255) -> ("error out"=w251:errorcluster)  [unwired: 5 in, 1 out]
                n286 = call <vilib>:"Clear Errors.vi"("error in (no error)"=w259) -> ()  [unwired: 5 in, 2 out]
                n287 = Enqueue Element(queue=w250, element="Stop", error in (no error)=w251) -> (error out=w249:errorcluster)  [unwired: 1 in, 2 out]
                n288 = call "ComunicacaoMedicao.vi"("error in"=w262, "Operação"=T9."FinalizarRotacao") -> ("error out"=w263:errorcluster)  [unwired: 7 in, 2 out]
                n289 = call <vilib>:"Clear Errors.vi"("error in (no error)"=w249) -> ()  [unwired: 5 in, 2 out]
                n290 = case shown="Error .." w263 {
                  selector: w263 -> [_ w270]
                  tunnel: w260 -> [w264 _]
                  frame No Error {
                    n291 = local write "Info"(w264) -> ()
                    n292 = Wait (ms)(milliseconds to wait=u32 2000) -> ()  [unwired: 1 out]
                  }
                  frame Error {
                    n293 = Unbundle By Name(w270) -> ("source"=w268:string)
                    n294 = Concatenate Strings("Erro na Comunicação com o inversor" ("Info"), "\r", w268) -> (w267:string)
                    n295 = local write "Info"(w267) -> ()
                  }
                }
              }
              frame "SetRampa" {
                n296 = local read "InfoContinuoRef"() -> (w271:T1)
                n297 = Unbundle By Name(w271) -> ("TempRampas"=w272:dbl)
                n298 = call "ComunicacaoMedicao.vi"("Palavra escrita"=w272, "Operação"=T10."TempoDesaceleração") -> ("error out"=w276:errorcluster)  [unwired: 7 in, 2 out]
                n299 = call "ComunicacaoMedicao.vi"("Palavra escrita"=w272, "Operação"=T10."TempoAceleracao") -> ("error out"=w277:errorcluster)  [unwired: 7 in, 2 out]
                n300 = Merge Errors(w277, w276) -> (w275:errorcluster)
                n301 = case shown="Error .." w275 {
                  selector: w275 -> [_ w282]
                  frame No Error {
                  }
                  frame Error {
                    n302 = Unbundle By Name(w282) -> ("source"=w280:string)
                    n303 = Concatenate Strings("Erro na Comunicação com o inversor" ("Info"), "\r", w280) -> (w279:string)
                    n304 = local write "Info"(w279) -> ()
                  }
                }
              }
              frame "SetVelocidade" {
                n305 = local read "InfoContinuoRef"() -> (w284:T1)
                n306 = Unbundle By Name(w284) -> ("PicoMax"=w285:dbl)
                n307 = call "ComunicacaoMedicao.vi"("Palavra escrita"=w285, "Operação"=T9."OndaContinua") -> ("error out"=w283:errorcluster)  [unwired: 7 in, 2 out]
                n308 = case shown="No Error" w283 {
                  selector: w283 -> [_ w291]
                  frame No Error {
                  }
                  frame Error {
                    n309 = Unbundle By Name(w291) -> ("source"=w289:string)
                    n310 = Concatenate Strings("Erro na Comunicação com o inversor" ("Info"), "\r", w289) -> (w288:string)
                    n311 = local write "Info"(w288) -> ()
                  }
                }
              }
              frame "ContinuaOnda" {
                n312 = local read "VelocidadeExaustor"() -> (w292:cluster{"X":dbl, "Y":dbl}[])
                n313 = local write "GraphCont"(w292) -> ()
                n314 = local read "TimeInicio"() -> (w293:u32)
                n315 = call "TimeStopTeste.vi"("TimeInicio"=w293) -> ("StopTeste"=w294:bool)  [unwired: 10 in]
                n316 = case shown="True" w294 {
                  selector: w294 -> [_ w304]
                  tunnel: w296 -> [w300 w303]
                  tunnel: w295 -> [w299 w302]
                  frame False {
                    n317 = Enqueue Element(queue=w299, element="ContinuaOnda", error in (no error)=w300) -> (error out=w298:errorcluster)  [unwired: 1 in, 2 out]
                    n318 = call <vilib>:"Clear Errors.vi"("error in (no error)"=w298) -> ()  [unwired: 5 in, 2 out]
                  }
                  frame True {
                    n319 = Flush Queue(queue=w302, error in (no error)=w303) -> (error out=w301:errorcluster)  [unwired: 2 out]
                    n320 = call <vilib>:"Clear Errors.vi"("error in (no error)"=w301) -> ()  [unwired: 5 in, 2 out]
                    n321 = property on="Stop" class="Bool (strict)"("Val(Sgnl)"=w304) -> ()  [unwired: 2 in, 2 out]
                  }
                }
              }
              frame "Senoidal" {
                n322 = global read "VariaveisParametros.vi" "TaxaTransmissãoDados"() -> (w307:dbl)
                n323 = local read "TimeNow"() -> (w314:u32)
                n324 = local read "TimeLast"() -> (w313:u32)
                n325 = Subtract(x=w314, y=w313) -> (x-y=w306:u32)
                n326 = Multiply(x=u32 1000 ("y"), y=w307) -> (x*y=w308:dbl)
                n327 = local read "TimeInicio"() -> (w305:u32)
                n328 = Greater Or Equal?(x=w306, y=w308) -> (x >= y?=w312:bool)
                n329 = case shown="True" w312 {
                  tunnel: [errorcluster {"status"=FALSE, "code"=0, "source"=""} ("error out") w344] -> w311
                  tunnel: w307 -> [_ w340]
                  tunnel: [w334 w338] -> _
                  tunnel: w306 -> [w334 w338]
                  tunnel: w305 -> [_ w337]
                  frame False {
                    n330 = Tick Count (ms)() -> (millisecond timer value=w335:u32)
                    n331 = local write "TimeNow"(w335) -> ()
                  }
                  frame True {
                    # "Acontece a cada 1s"
                    n332 = Tick Count (ms)() -> (millisecond timer value=w345:u32)
                    n333 = global read "VariaveisParametros.vi" "InfoInSenoide"() -> (w341:T11)
                    n334 = local write "TimeNow"(w345) -> ()
                    n335 = local write "TimeLast"(w345) -> ()
                    n336 = call "CalculoOndaSenoide.vi"("TimeInicio"=w337, "Taxa"=w340, "InfoInSenoide"=w341, "GraphSenoide"="GraphSenoide") -> ("XY Graph"=w339:cluster{"X":dbl, "Y":dbl}[])  [unwired: 7 in]
                    n337 = Delete From Array(array=w339) -> (deleted portion=w343:cluster{"X":dbl, "Y":dbl})  [unwired: 2 in, 1 out]
                    n338 = local write "GraphSenoide"(w339) -> ()
                    n339 = stacked-sequence {
                      seq-local: [w346 _ _] -> [_ _ w352]
                      tunnel: [_ w349 _] -> w344
                      tunnel: w343 -> [_ w348 _]
                      tunnel: [_ _ w351] -> _
                      frame #0 {
                        n340 = Tick Count (ms)() -> (millisecond timer value=w346:u32)
                      }
                      frame #1 {
                        n341 = Unbundle By Name(w348) -> ("Y"=w350:dbl)
                        n342 = call "ComunicacaoMedicao.vi"("Palavra escrita"=w350, "Operação"=T9."OndaSenoide") -> ("error out"=w349:errorcluster)  [unwired: 7 in, 2 out]
                      }
                      frame #2 {
                        n343 = Tick Count (ms)() -> (millisecond timer value=w353:u32)
                        n344 = Subtract(x=w353, y=w352) -> (x-y=w351:u32)
                      }
                    }
                  }
                }
                n345 = call "TimeStopTeste.vi"("TimeInicio"=w305) -> ("StopTeste"=w310:bool)  [unwired: 10 in]
                n346 = case shown="False" w310 {
                  selector: w310 -> [_ w333]
                  tunnel: w316 -> [w319 w332]
                  tunnel: w315 -> [w318 w331]
                  tunnel: w311 -> [w317 _]
                  frame False {
                    n347 = case shown="No Error" w317 {
                      selector: w317 -> [_ w325]
                      tunnel: w319 -> [w323 _]
                      tunnel: w318 -> [w322 _]
                      frame No Error {
                        n348 = Enqueue Element(queue=w322, element="Senoidal", error in (no error)=w323) -> (error out=w321:errorcluster)  [unwired: 1 in, 2 out]
                        n349 = call <vilib>:"Clear Errors.vi"("error in (no error)"=w321) -> ()  [unwired: 5 in, 2 out]
                      }
                      frame Error {
                        n350 = Unbundle By Name(w325) -> ("source"=w329:string)
                        n351 = property on="Stop" class="Bool (strict)"("Val(Sgnl)"=TRUE ("Visible")) -> ()  [unwired: 2 in, 2 out]
                        n352 = Concatenate Strings("Erro na Comunicação com o inversor" ("Info"), "\r", w329) -> (w328:string)
                        n353 = local write "Info"(w328) -> ()
                      }
                    }
                  }
                  frame True {
                    n354 = Flush Queue(queue=w331, error in (no error)=w332) -> (error out=w330:errorcluster)  [unwired: 2 out]
                    n355 = call <vilib>:"Clear Errors.vi"("error in (no error)"=w330) -> ()  [unwired: 5 in, 2 out]
                    n356 = property on="Stop" class="Bool (strict)"("Val(Sgnl)"=w333) -> ()  [unwired: 2 in, 2 out]
                  }
                }
              }
              frame "Pontos" {
                n357 = global read "VariaveisParametros.vi" "TempoEntrePontos"() -> (w355:dbl)
                n358 = local read "TimeNow"() -> (w362:u32)
                n359 = local read "TimeLast"() -> (w361:u32)
                n360 = Subtract(x=w362, y=w361) -> (x-y=w360:u32)
                n361 = Multiply(x=u32 1000 ("y"), y=w355) -> (x*y=w356:dbl)
                n362 = Greater Or Equal?(x=w360, y=w356) -> (x >= y?=w359:bool)
                n363 = case shown="True" w359 {
                  tunnel: [errorcluster {"status"=FALSE, "code"=0, "source"=""} ("error out") w393] -> w358
                  tunnel: w355 -> [_ w388]
                  tunnel: [FALSE ("Stop") w386] -> w354
                  frame False {
                    n364 = Tick Count (ms)() -> (millisecond timer value=w383:u32)
                    n365 = local write "TimeNow"(w383) -> ()
                  }
                  frame True {
                    # "Acontece a cada 1s"
                    n366 = local read "TimeInicio"() -> (w385:u32)
                    n367 = global read "VariaveisParametros.vi" "Pontos"() -> (w387:dbl[])
                    n368 = call "CalculoOndaPontos.vi"("TimeInicio"=w385, "TempoEntrePontos"=w388, "Pontos"=w387, "GraphPontos"="GraphPontos") -> ("Stop"=w386:bool, "XY Graph"=w390:cluster{"X":dbl, "Y":dbl}[])  [unwired: 6 in]
                    n369 = Delete From Array(array=w390) -> (deleted portion=w392:cluster{"X":dbl, "Y":dbl})  [unwired: 2 in, 1 out]
                    n370 = local write "GraphPontos"(w390) -> ()
                    n371 = Tick Count (ms)() -> (millisecond timer value=w395:u32)
                    n372 = Unbundle By Name(w392) -> ("Y"=w394:dbl)
                    n373 = local write "TimeNow"(w395) -> ()
                    n374 = local write "TimeLast"(w395) -> ()
                    n375 = call "ComunicacaoMedicao.vi"("Palavra escrita"=w394, "Operação"=T9."OndaPontos") -> ("error out"=w393:errorcluster)  [unwired: 7 in, 2 out]
                  }
                }
                n376 = case shown="True" w354 {
                  selector: w354 -> [_ w381]
                  tunnel: w364 -> [w367 w380]
                  tunnel: w363 -> [w366 w379]
                  tunnel: w358 -> [w365 _]
                  frame False {
                    n377 = case shown="No Error" w365 {
                      selector: w365 -> [_ w373]
                      tunnel: w367 -> [w371 _]
                      tunnel: w366 -> [w370 _]
                      frame No Error {
                        n378 = Enqueue Element(queue=w370, element="Pontos", error in (no error)=w371) -> (error out=w369:errorcluster)  [unwired: 1 in, 2 out]
                        n379 = call <vilib>:"Clear Errors.vi"("error in (no error)"=w369) -> ()  [unwired: 5 in, 2 out]
                      }
                      frame Error {
                        n380 = Unbundle By Name(w373) -> ("source"=w377:string)
                        n381 = property on="Stop" class="Bool (strict)"("Val(Sgnl)"=TRUE ("Visible")) -> ()  [unwired: 2 in, 2 out]
                        n382 = Concatenate Strings("Erro na Comunicação com o inversor" ("Info"), "\r", w377) -> (w376:string)
                        n383 = local write "Info"(w376) -> ()
                      }
                    }
                  }
                  frame True {
                    n384 = Flush Queue(queue=w379, error in (no error)=w380) -> (error out=w378:errorcluster)  [unwired: 2 out]
                    n385 = call <vilib>:"Clear Errors.vi"("error in (no error)"=w378) -> ()  [unwired: 5 in, 2 out]
                    n386 = property on="Stop" class="Bool (strict)"("Val(Sgnl)"=w381) -> ()  [unwired: 2 in, 2 out]
                  }
                }
              }
            }
          }
          frame Error {
          }
        }
      }
      n387 = while {
        tunnel: w94 -> [w110]
        tunnel: w95 -> [w109]
        stop <- w111 stop-if-true
        # "Leitura de sinais"
        n388 = Dequeue Element(queue=w109, error in (no error)=w110) -> (queue out=w108:refnum<queue>, element=w112:string, error out=w113:errorcluster)  [unwired: 1 in, 1 out]
        n389 = case shown="No Error" w113 {
          selector: w113 -> [w115 _]
          tunnel: w112 -> [w116 _]
          tunnel: [_ TRUE] -> w111
          tunnel: w108 -> [w114 _]
          frame No Error {
            n390 = case shown="\"Iniciar\"" w116 {
              tunnel: w115 -> [_ w123 w168]
              tunnel: w114 -> [_ w122 w167]
              frame "False", Default {
              }
              frame "Iniciar" {
                n391 = local read "TimeNowMed"() -> (w121:u32)
                n392 = local read "TimeLastMed"() -> (w120:u32)
                n393 = local read "TimeAquisicao"() -> (w117:i32)
                n394 = Enqueue Element(queue=w122, element="Iniciar", error in (no error)=w123) -> (error out=w124:errorcluster)  [unwired: 1 in, 2 out]
                n395 = call <vilib>:"Clear Errors.vi"("error in (no error)"=w124) -> ()  [unwired: 5 in, 2 out]
                n396 = Subtract(x=w121, y=w120) -> (x-y=w119:u32)
                n397 = Greater Or Equal?(x=w119, y=w117) -> (x >= y?=w118:bool)
                n398 = case shown="True" w118 {
                  frame False {
                    n399 = Tick Count (ms)() -> (millisecond timer value=→"TimeNowMed":u32)
                  }
                  frame True {
                    n400 = stacked-sequence {
                      frame #0 {
                      }
                      frame #1 {
                        n401 = local read "ListaMedicoes"() -> (w127:string[][])
                        n402 = for {
                          tunnel: w127 -> [w133] mode=indexing
                          n403 = Index Array(array=w133, index=3) -> (element=w132:string)
                          n404 = Decimal String To Number(string=w132) -> (number=w131:i32)  [unwired: 2 in, 1 out]
                          n405 = local read "TimeInicio"() -> (w129:u32)
                          n406 = call "TempoAtual.vi"("TimeInicio"=w129) -> ("TempoAtual"=w128:dbl)  [unwired: 10 in]
                          n407 = case shown="1" w131 {
                            tunnel: w128 -> [_ w134 w140 w146 w152]
                            frame 0, Default {
                            }
                            frame 1 {
                              n408 = global read "VariaveisTaskMedicao.vi" "TensaoAeroGerador"() -> (w135:dbl)
                              n409 = local read "TensaoAero"() -> (w136:cluster{"X":dbl, "Y":dbl}[])
                              n410 = Bundle By Name(cluster=cluster{"X":dbl, "Y":dbl} {"X"=0.0, "Y"=0.0} ("new element/subarray"), "X"=w134, "Y"=w135) -> (w138:cluster{"X":dbl, "Y":dbl})
                              n411 = Insert Into Array(array=w136, new element=w138) -> (→"TensaoAero":cluster{"X":dbl, "Y":dbl}[])  [unwired: 1 in]
                            }
                            frame 2 {
                              n412 = global read "VariaveisTaskMedicao.vi" "CorrenteAeroGerador"() -> (w141:dbl)
                              n413 = local read "CorrenteAero"() -> (w142:cluster{"X":dbl, "Y":dbl}[])
                              n414 = Bundle By Name(cluster=cluster{"X":dbl, "Y":dbl} {"X"=0.0, "Y"=0.0} ("new element/subarray"), "X"=w140, "Y"=w141) -> (w144:cluster{"X":dbl, "Y":dbl})
                              n415 = Insert Into Array(array=w142, new element=w144) -> (→"CorrenteAero":cluster{"X":dbl, "Y":dbl}[])  [unwired: 1 in]
                            }
                            frame 3 {
                              n416 = local read "Anemometro1"() -> (w148:cluster{"X":dbl, "Y":dbl}[])
                              n417 = global read "VariaveisTaskMedicao.vi" "Anemômetro1"() -> (w147:dbl)
                              n418 = Bundle By Name(cluster=cluster{"X":dbl, "Y":dbl} {"X"=0.0, "Y"=0.0} ("new element/subarray"), "X"=w146, "Y"=w147) -> (w150:cluster{"X":dbl, "Y":dbl})
                              n419 = Insert Into Array(array=w148, new element=w150) -> (→"Anemometro1":cluster{"X":dbl, "Y":dbl}[])  [unwired: 1 in]
                            }
                            frame 4 {
                              n420 = local read "Anemometro2"() -> (w154:cluster{"X":dbl, "Y":dbl}[])
                              n421 = global read "VariaveisTaskMedicao.vi" "Anemômetro2"() -> (w153:dbl)
                              n422 = Bundle By Name(cluster=cluster{"X":dbl, "Y":dbl} {"X"=0.0, "Y"=0.0} ("new element/subarray"), "X"=w152, "Y"=w153) -> (w156:cluster{"X":dbl, "Y":dbl})
                              n423 = Insert Into Array(array=w154, new element=w156) -> (→"Anemometro2":cluster{"X":dbl, "Y":dbl}[])  [unwired: 1 in]
                            }
                          }
                        }
                      }
                      frame #2 {
                        n424 = local read "VelocidadeExaustor"() -> (w161:cluster{"X":dbl, "Y":dbl}[])
                        n425 = local read "TimeInicio"() -> (w159:u32)
                        n426 = call "ComunicacaoMedicao.vi"("Operação"=T8."VelocidadeExaustor") -> ("Valor"=w160:dbl)  [unwired: 8 in, 2 out]
                        n427 = call "TempoAtual.vi"("TimeInicio"=w159) -> ("TempoAtual"=w158:dbl)  [unwired: 10 in]
                        n428 = Bundle By Name(cluster=cluster{"X":dbl, "Y":dbl} {"X"=0.0, "Y"=0.0} ("new element/subarray"), "X"=w158, "Y"=w160) -> (w162:cluster{"X":dbl, "Y":dbl})
                        n429 = Insert Into Array(array=w161, new element=w162) -> (→"VelocidadeExaustor":cluster{"X":dbl, "Y":dbl}[])  [unwired: 1 in]
                      }
                      frame #3 {
                        n430 = Tick Count (ms)() -> (millisecond timer value=w166:u32)
                        n431 = local write "TimeNowMed"(w166) -> ()
                        n432 = local write "TimeLastMed"(w166) -> ()
                      }
                    }
                  }
                }
              }
              frame "Stop" {
                n433 = Flush Queue(queue=w167, error in (no error)=w168) -> (error out=w169:errorcluster)  [unwired: 2 out]
                n434 = call <vilib>:"Clear Errors.vi"("error in (no error)"=w169) -> ()  [unwired: 5 in, 2 out]
              }
            }
          }
          frame Error {
          }
        }
      }
      n435 = Release Queue(queue=w100, error in (no error)=w102) -> (error out=w97:errorcluster)  [unwired: 1 in, 2 out]
      n436 = Release Queue(queue=w95, error in (no error)=w97) -> (error out=w96:errorcluster)  [unwired: 1 in, 2 out]
      n437 = call <vilib>:"Clear Errors.vi"("error in (no error)"=w96) -> ()  [unwired: 5 in, 2 out]
    }
  }
